vi "BNT_DAQmx-Content.vi"() -> (0 "CS++Classes & Messages":T1(array[cluster]))   [LabVIEW 2020]
doc: "Place actor and class constants that should be included included in the COMPACT application on the blockdiagramm."
uses:
  <vilib>/ActorFramework/Message/Message.lvclass
  BNT_DAQmx-MCSV-AIAvg/BNT_DAQmx-MCSV-AIAvg.lvclass
  C:/Users/holge/Documents/LVP/BNT/PGC/Packages/BNT_DAQmx/BNT_DAQmx-MCSV/BNT_DAQmx-MCSV.lvclass
  BNT_DAQmx-MCSV-DOPWM/BNT_DAQmx-MCSV-DOPWM.lvclass
  BNT_DAQmx_MCSV-Ctr2Freq/BNT_DAQmx-MCSV-Ctr2Freq.lvclass
  BNT_DAQmx-MCSV-TC/BNT_DAQmx-MCSV-TC.lvclass
  BNT_DAQmx-MCSV-RTD/BNT_DAQmx-MCSV-RTD.lvclass
  BNT_DAQmx-MCSV/BNT_DAQmx-MCSV.lvclass
  C:/Users/holge/Documents/LVP/BNT/PGC/Packages/CSPP_Core/Actors/CSPP_BaseActor/CSPP_BaseActor.lvclass
  CSPP_Core/Actors/CSPP_BaseActor/CSPP_BaseActor.lvclass
panel:
  # "Place actor and class constants on the blockdiagramm."
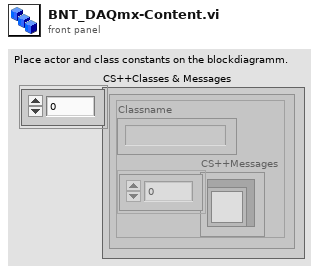
[diagram p1: front panel]
types:
  T1 = cluster{"Classname":string, "CS++Messages":refnum<class "Message.lvclass">[]}[]
  T2 = cluster{"class name":string, "CSPP_Messages":refnum<class "Message.lvclass">[]}
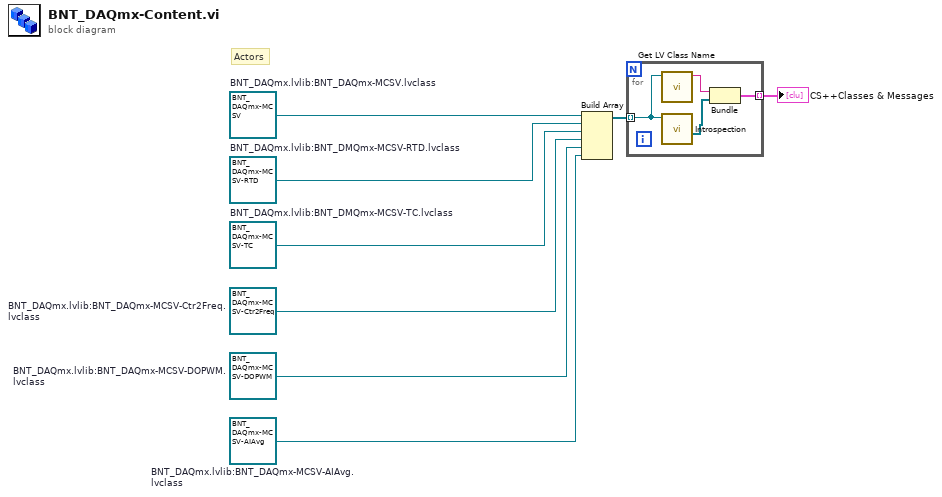
[diagram p0: block diagram]
diagram:
  w1 = refnum<class "BNT_DAQmx-MCSV-AIAvg.lvclass"> refnum  # BNT_DAQmx.lvlib:BNT_DAQmx-MCSV-AIAvg.lvclass
  w2 = refnum<class "BNT_DAQmx-MCSV-DOPWM.lvclass"> refnum  # BNT_DAQmx.lvlib:BNT_DAQmx-MCSV-DOPWM.lvclass
  w3 = refnum<class "BNT_DAQmx-MCSV-Ctr2Freq.lvclass"> refnum  # BNT_DAQmx.lvlib:BNT_DAQmx-MCSV-Ctr2Freq.lvclass
  w5 = refnum<class "BNT_DAQmx-MCSV-TC.lvclass"> refnum  # BNT_DAQmx.lvlib:BNT_DMQmx-MCSV-TC.lvclass
  w6 = refnum<class "BNT_DAQmx-MCSV-RTD.lvclass"> refnum  # BNT_DAQmx.lvlib:BNT_DMQmx-MCSV-RTD.lvclass
  w7 = refnum<class "BNT_DAQmx-MCSV.lvclass"> refnum  # BNT_DAQmx.lvlib:BNT_DAQmx-MCSV.lvclass
  # "Actors"
  n1 = Build Array(w7, w6, w5, w3, w2, w1) -> (w8:refnum<class "BNT_DAQmx-MCSV.lvclass">[])
  n2 = for {
    tunnel: w8 -> [w12] mode=indexing
    tunnel: [w10] -> w4 mode=indexing
    n3 = call <vilib>:"Get LV Class Name.vi"("object"=w12) -> ("class name"=w11:string)  [unwired: 9 in, 1 out]
    n4 = call "Introspection.vi"("CSPP_BaseActor in"=w12) -> ("CSPP_Messages"=w9:refnum<class "Message.lvclass">[])  [unwired: 7 in, 3 out]
    n5 = Bundle("class name"=w11, "CSPP_Messages"=w9) -> (w10:T2)  [unwired: 1 in]
  }
  "CS++Classes & Messages" <- w4
